vi "Set TestStand Icon.vi"(7 "VI Reference":refnum<vi>, 8 "Error In":errorcluster, 11 "Context":refnum<k7>) -> (0 "Error Out":errorcluster)   [LabVIEW 2021, in "Seq Edit Quick Drop.lvlib"]
uses:
  Seq Edit Quick Drop.lvlib
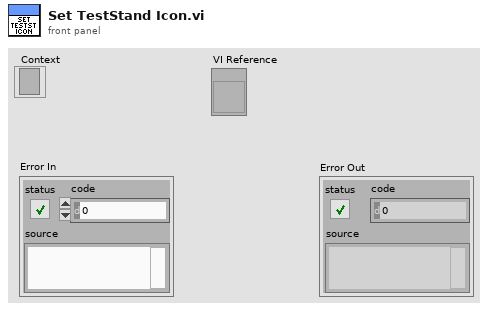
[diagram p1: front panel]
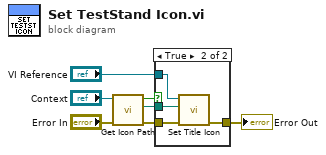
[diagram p0: block diagram]
diagram:
  n1 = call "Get Icon Path.vi"("Error In"="Error In", "Context"="Context") -> ("Error Out"=w7:errorcluster, "Path"=w6:path, "Found?"=w5:bool)  [unwired: 7 in]
  n2 = case shown="True" w5 {
    tunnel: w7 -> [w8 w12]
    tunnel: w6 -> [_ w11]
    tunnel: [w8 w10] -> w2
    tunnel: "VI Reference" -> [_ w9]
    frame False {
    }
    frame True {
      n3 = call "Set Title Icon.vi"("Error In"=w12, "Icon Path"=w11, "VI Reference"=w9) -> ("Error Out"=w10:errorcluster)  [unwired: 8 in]
    }
  }
  "Error Out" <- w2
